vi "Prelabs_Consolidated.vi"() -> ()   [LabVIEW 2017]
uses:
  <vilib>/Analysis/2dsp.llb/Real FFT.vi
  <vilib>/Analysis/2dsp.llb/Decimate (single shot, DBL).vi
  <vilib>/Utility/file.llb/Read Delimited Spreadsheet (DBL).vi
  <vilib>/Analysis/3filter.llb/Butterworth Filter (DBL).vi
  <vilib>/Analysis/NI_AALBase.lvlib
  <vilib>/Analysis/NI_AALPro.lvlib
panel:
  in  "High Cutoff":dbl=20.0
  in  "Resample factor":i32=2
  in  "Amplitude":dbl=0.3
  in  "Resample?":bool
  in  "Apply filter?":bool
  in  "Add sine wave noise?":bool
  in  "Add white noise?":bool
  out "Time Domain Signal":cluster{i32, dbl, dbl[]}(graph)={0, 0.008, []}
  in  "Sine wave\nfrequency":dbl=60.0
  in  "Low Cutoff":dbl=20.0
  in  "Amplitude":dbl=0.01
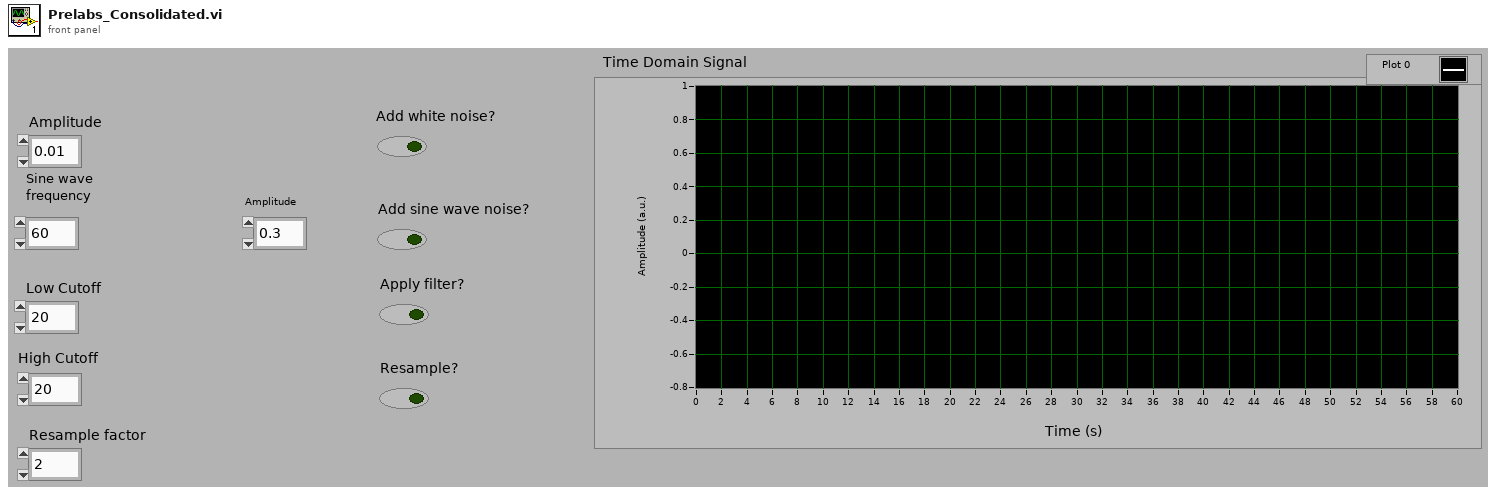
[diagram p1: front panel]
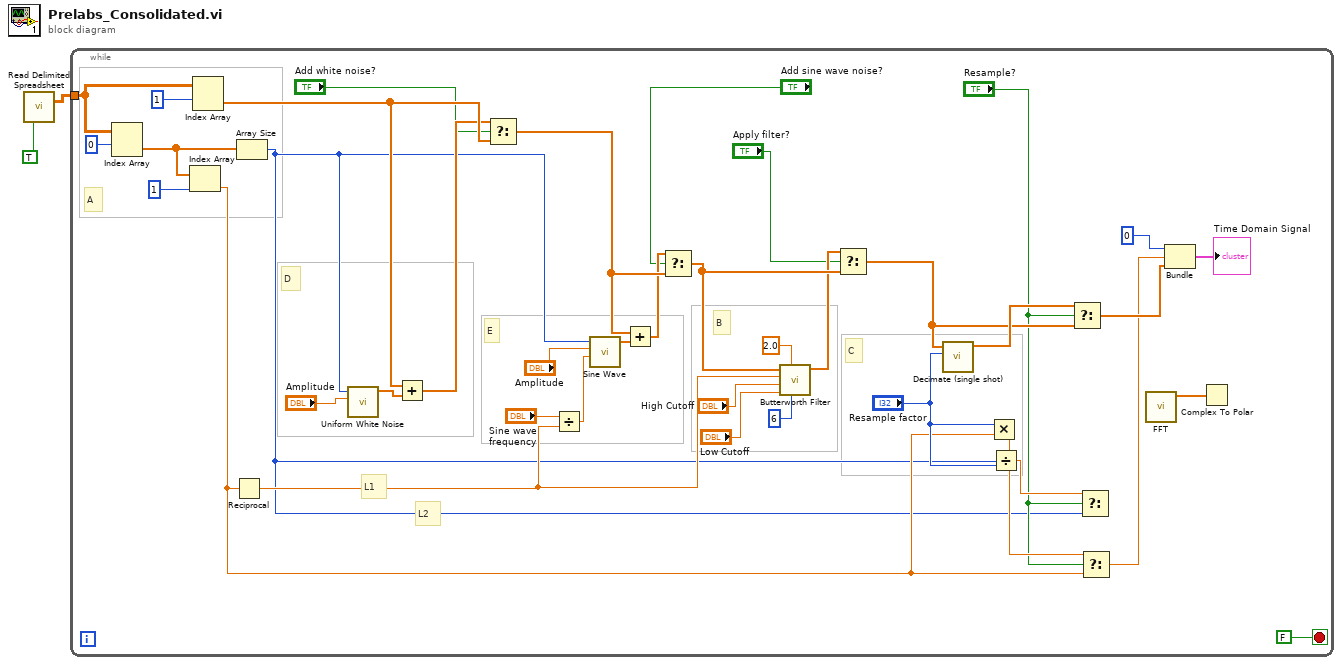
[diagram p0: block diagram]
diagram:
  n1 = call-poly <vilib>:"Read Delimited Spreadsheet.vi"("transpose? (F)"=TRUE ("Boolean")) -> ("all rows"=w1:dbl[][])  [unwired: 9 in, 5 out]
  n2 = while {
    tunnel: w1 -> [w21]
    stop <- FALSE stop-if-true
    # "L2"
    # "L1"
    # "C"
    # "B"
    # "E"
    # "D"
    # "A"
    n3 = Index Array(array=w21, index (row)=0) -> (element=w17:dbl[])  [unwired: 1 in]
    n4 = Index Array(array=w17, index=1) -> (element=w11:dbl)
    n5 = Index Array(array=w21, index (row)=1) -> (element=w33:dbl[])  [unwired: 1 in]
    n6 = Reciprocal(x=w11) -> (1/x=w18:dbl)
    n7 = Array Size(array=w17) -> (size(s)=w7:i32)
    n8 = call <vilib>:"Uniform White Noise.vi"("amplitude"="Amplitude", "samples"=w7) -> ("uniform white noise"=w5:dbl[])  [unwired: 8 in, 1 out]
    n9 = Add(x=w33, y=w5) -> (x+y=w32:dbl[])
    n10 = Select(t=w32, s="Add white noise?", f=w33) -> (s? t:f=w30:dbl[])
    n11 = Divide(x="Sine wave\nfrequency", y=w18) -> (x/y=w37:dbl)
    n12 = call <vilib>:"Sine Wave.vi"("samples"=w7, "amplitude"="Amplitude", "frequency"=w37) -> ("sine wave"=w35:dbl[])  [unwired: 2 in, 2 out]
    n13 = Add(x=w30, y=w35) -> (x+y=w29:dbl[])
    n14 = Select(t=w29, s="Add sine wave noise?", f=w30) -> (s? t:f=w27:dbl[])
    n15 = call-poly <vilib>:"Butterworth Filter.vi"("order"=6 ("Filter order"), "filter type"=2.0 ("Filter Type"), "low cutoff freq: fl"="Low Cutoff", "high cutoff freq: fh"="High Cutoff", "sampling freq: fs"=w18, "X"=w27) -> ("Filtered X"=w26:dbl[])  [unwired: 1 in, 2 out]
    n16 = Select(t=w26, s="Apply filter?", f=w27) -> (s? t:f=w23:dbl[])
    n17 = call-poly <vilib>:"Decimate (single shot).vi"("decimating factor"="Resample factor", "X"=w23) -> ("Decimated Array"=w24:dbl[])  [unwired: 1 in, 8 out]
    n18 = Multiply(x="Resample factor", y=w11) -> (x*y=w15:dbl)
    n19 = Divide(x=w7, y="Resample factor") -> (x/y=w13:dbl)
    n20 = Select(t=w24, s="Resample?", f=w23) -> (s? t:f=w10:dbl[])
    n21 = Select(t=w13, s="Resample?", f=w7) -> ()  [unwired: 1 out]
    n22 = Select(t=w15, s="Resample?", f=w11) -> (s? t:f=w8:dbl)
    n23 = call-poly <vilib>:"FFT.vi"() -> ("FFT {X}"=w3:cdb[])  [unwired: 3 in, 8 out]
    n24 = Bundle(0, "Numeric"=w8, "all rows"=w10) -> (→"Time Domain Signal":cluster{i32, "Numeric":dbl, "all rows":dbl[]})  [unwired: 1 out]
    n25 = Complex To Polar(r * e^(i*theta)=w3) -> ()  [unwired: 2 out]
  }
